vi "Search Song Library.vi"(8 "error in (no error)":errorcluster, 10 "Search String":string, 11 "MusicManagerActor in":refnum<class "MusicManagerActor.lvclass">) -> (0 "error out":errorcluster, 3 "MusicManagerActor out":refnum<class "MusicManagerActor.lvclass">)   [LabVIEW 2015, in "MusicManagerActor.lvlib" / "MusicManagerActor.lvclass"]
uses:
  MusicManagerActor.lvclass
  MusicManagerActor.lvclass/MusicManagerActor.ctl
  file/MusicElement/MusicElement.lvclass/MusicElement.ctl
  file/MusicElement/Song/Song.lvclass/Song.ctl
  file/MusicElement/Song/Song.lvclass
  SongBrowserActor/SongBrowserActor Messages/Display Song Library Msg/Display Song Library Msg.lvclass
  file/MusicElement/MusicElement.lvclass
  file/MusicElement/MusicElementLibrary/MusicLibrary/MusicLibrary.lvclass
  file/MusicElement/MusicElementLibrary/SongLibrary/SongLibrary.lvclass
  SongQueueActor/SongQueueActor Messages/Set Visibility Of Queue List Msg/Set Visibility Of Queue List Msg.lvclass
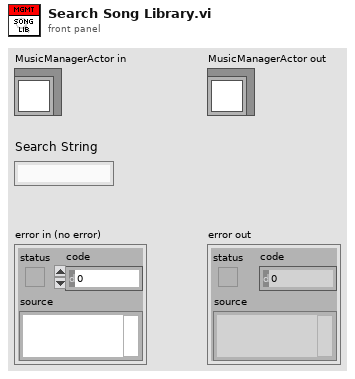
[diagram p1: front panel]
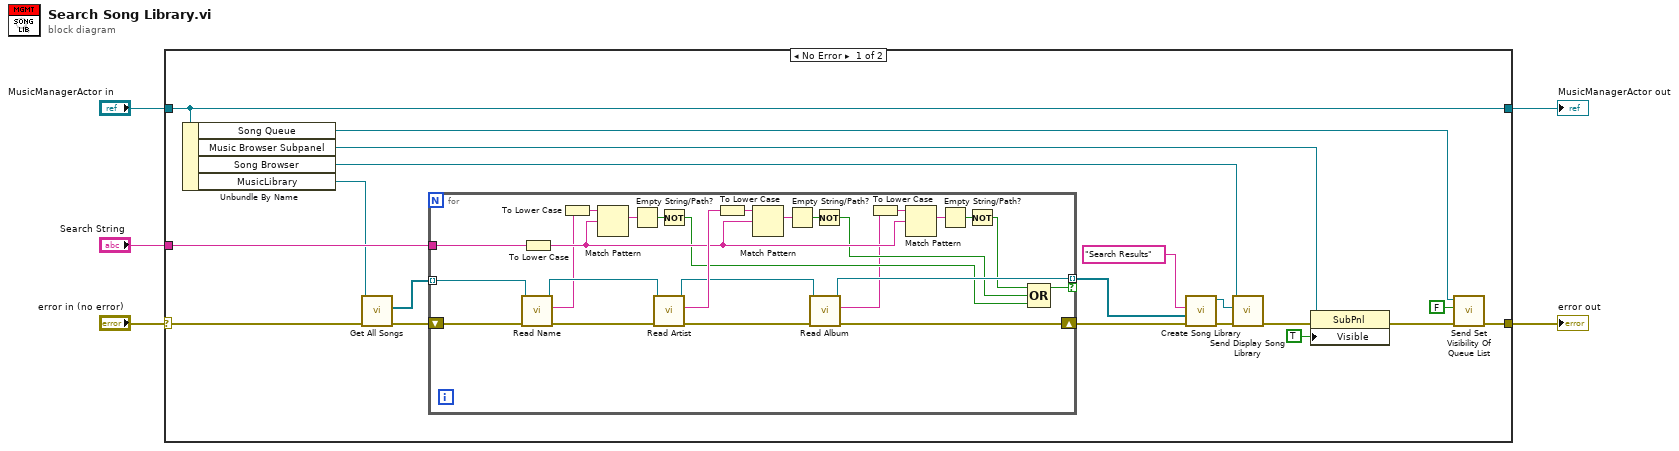
[diagram p0: block diagram]
diagram:
  n1 = case shown="No Error" "error in (no error)" {
    selector: "error in (no error)" -> [w21 w52]
    tunnel: [w8 w52] -> w4
    tunnel: [w24 w51] -> w2
    tunnel: "MusicManagerActor in" -> [w24 w51]
    tunnel: "Search String" -> [w22 _]
    frame No Error {
      n2 = Unbundle By Name(w24) -> ("Song Queue"=w6:refnum<class "Message Enqueuer.lvclass">, "Music Browser Subpanel"=w7:refnum<vi>, "Song Browser"=w23:refnum<class "Message Enqueuer.lvclass">, "MusicLibrary"=w20:refnum<class "MusicLibrary.lvclass">)
      n3 = call "Get All Songs.vi"("error in (no error)"=w21, "MusicLibrary in"=w20) -> ("error out"=w19:errorcluster, "Songs"=w18:refnum<class "Song.lvclass">[])  [unwired: 7 in, 1 out]
      n4 = for {
        shift-right: [w35] -> w17
        shift-left: w19 -> [w29]
        tunnel: w18 -> [w27] mode=indexing
        tunnel: w22 -> [w48]
        tunnel: [w36] -> w13 mode=indexing if=w31
        n5 = call "Read Name.vi"("error in (no error)"=w29, "MusicElement in"=w27) -> ("error out"=w28:errorcluster, "Name"=w25:string, "MusicElement out"=w26:refnum<class "Song.lvclass">)  [unwired: 7 in]
        n6 = To Lower Case(string=w48) -> (all lower case string=w39:string)
        n7 = To Lower Case(string=w25) -> (all lower case string=w47:string)
        n8 = Match Pattern(string=w47, regular expression=w39) -> (match substring=w50:string)  [unwired: 1 in, 3 out]
        n9 = Empty String/Path?(string/path=w50) -> (empty?=w49:bool)
        n10 = call "Read Artist.vi"("error in (no error)"=w28, "Song in"=w26) -> ("error out"=w38:errorcluster, "Artist"=w40:string, "Song out"=w37:refnum<class "Song.lvclass">)  [unwired: 7 in]
        n11 = Not(x=w49) -> (.not. x?=w32:bool)
        n12 = To Lower Case(string=w40) -> (all lower case string=w46:string)
        n13 = Match Pattern(string=w46, regular expression=w39) -> (match substring=w44:string)  [unwired: 1 in, 3 out]
        n14 = Empty String/Path?(string/path=w44) -> (empty?=w45:bool)
        n15 = call "Read Album.vi"("error in (no error)"=w38, "Song in"=w37) -> ("error out"=w35:errorcluster, "Album"=w30:string, "Song out"=w36:refnum<class "Song.lvclass">)  [unwired: 7 in]
        n16 = Not(x=w45) -> (.not. x?=w33:bool)
        n17 = To Lower Case(string=w30) -> (all lower case string=w41:string)
        n18 = Match Pattern(string=w41, regular expression=w39) -> (match substring=w43:string)  [unwired: 1 in, 3 out]
        n19 = Empty String/Path?(string/path=w43) -> (empty?=w42:bool)
        n20 = Not(x=w42) -> (.not. x?=w34:bool)
        n21 = Compound Arithmetic op=OR(w34, w33, w32) -> (w31:bool)
      }
      n22 = call "Create Song Library.vi"("error in (no error)"=w17, "Songs"=w13, "Name"="Search Results") -> ("error out"=w16:errorcluster, "SongLibrary out"=w15:refnum<class "SongLibrary.lvclass">)  [unwired: 7 in]
      n23 = call "Send Display Song Library.vi"("error in (no error)"=w16, "Song Library"=w15, "Message Enqueuer in"=w23) -> ("error out"=w9:errorcluster)  [unwired: 7 in, 1 out]
      n24 = property class="SubPnl"(reference=w7, error in=w9, "Visible"=TRUE) -> (error out=w10:errorcluster)  [unwired: 1 out]
      n25 = call "Send Set Visibility Of Queue List.vi"("error in (no error)"=w10, "Visible"=FALSE, "Message Enqueuer in"=w6) -> ("error out"=w8:errorcluster)  [unwired: 7 in, 1 out]
    }
    frame Error {
    }
  }
  "error out" <- w4
  "MusicManagerActor out" <- w2
